vi "practica3.vi"() -> ()   [LabVIEW 2020]
panel:
  out "Filtered Signal 2":dynamicdata(graph) caption="Filtered Signal"
  out "Filtered Signal":dynamicdata(graph)
  out "Data":dynamicdata(graph)
  in  "stop":bool
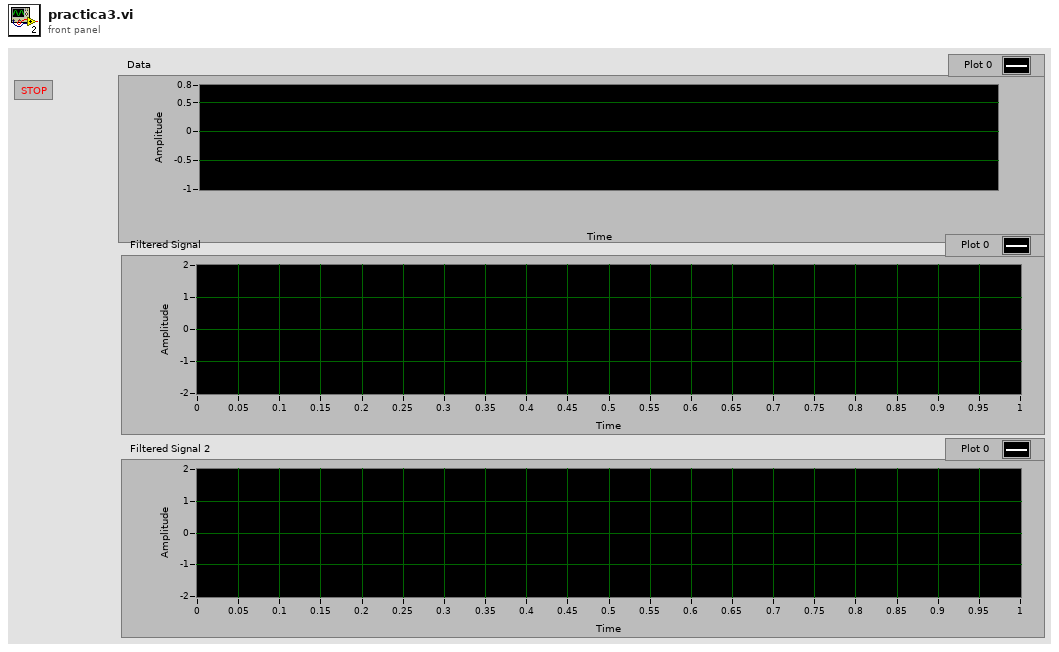
[diagram p1: front panel]
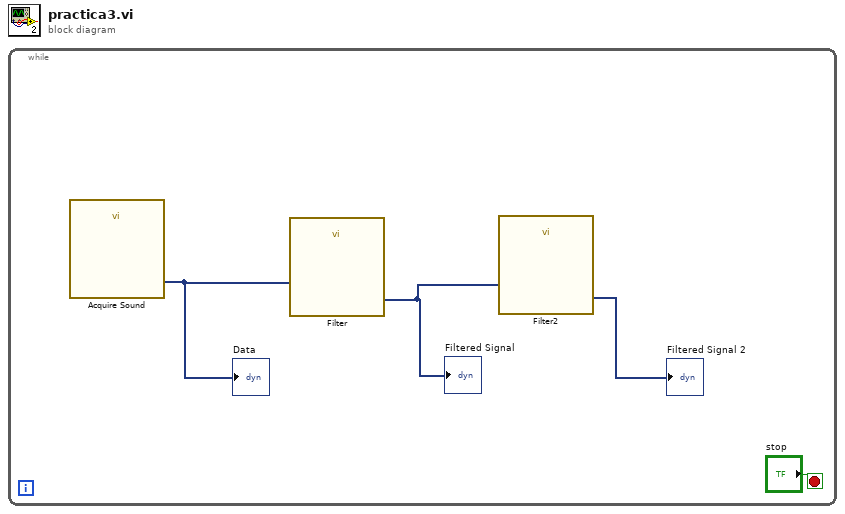
[diagram p0: block diagram]
diagram:
  n1 = while {
    stop <- "stop" stop-if-true
    n2 = call "Acquire Sound"() -> ("Data"=w3:dynamicdata)  [unwired: 18 in, 1 out]
    "Data" <- w3
    n3 = call "Filter"("Signal"=w3) -> ("Filtered Signal"=w2:dynamicdata)  [unwired: 9 in, 1 out]
    "Filtered Signal" <- w2
    n4 = call "Filter2"("Signal"=w2) -> ("Filtered Signal"=→"Filtered Signal 2":dynamicdata)  [unwired: 9 in, 1 out]
  }
